vi "Close Pipe (writer).vi"(8 "error in (no error)":errorcluster, 11 "pipe in":refnum<data-value>) -> (0 "error out":errorcluster, 3 "pathname out":string)   [LabVIEW 2013, in "Linux RT IPC.lvlib" / "Pipes.lvlib" / "Unix Pipe Writer.lvclass"]
doc: "This VI closes the endpoint, preventing the endpoint from reading from or writing to the pipe. This does not remove the pipe from the filesystem, so other endpoints can continue to use the pipe."
uses:
  Unix Pipe Writer.lvclass
  Unix Pipe/Unix Pipe.lvclass/Unix Pipe.ctl
  C/C.lvlib
  Unix Pipe/Unix Pipe.lvclass
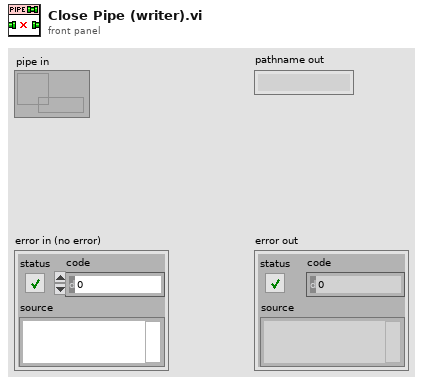
[diagram p1: front panel]
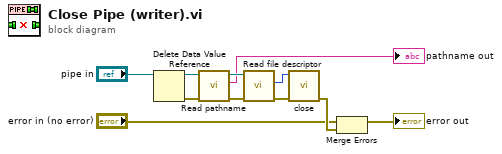
[diagram p0: block diagram]
diagram:
  n1 = Delete Data Value Reference(data value reference="pipe in") -> (data value=w3:refnum<class "Unix Pipe Writer.lvclass">, error out=w5:errorcluster)  [unwired: 1 in]
  n2 = call "Read pathname.vi"("error in (no error)"=w5, "Unix Pipe in"=w3) -> ("error out"=w4:errorcluster, "pathname"=→"pathname out":string, "Unix Pipe out"=w2:refnum<class "Unix Pipe Writer.lvclass">)  [unwired: 7 in]
  n3 = call "Read file descriptor.vi"("error in (no error)"=w4, "Unix Pipe in"=w2) -> ("error out"=w10:errorcluster, "file descriptor"=w9:i32)  [unwired: 7 in, 1 out]
  n4 = call "close.vi"("error in (no error)"=w10, "file descriptor in"=w9) -> ("error out"=w8:errorcluster)  [unwired: 9 in]
  n5 = Merge Errors("error in (no error)", w8) -> (→"error out":errorcluster)
